vi "Write VariableGroupRingRef.vi"(8 "error in (no error)":errorcluster, 10 "VariableGroupRingRef":refnum<vi>, 11 "VMUI in":refnum<class "VMUI.lvclass">) -> (0 "error out":errorcluster, 3 "VMUI out":refnum<class "VMUI.lvclass">)   [LabVIEW 2013, in "VMUI.lvclass"]
uses:
  VMUI.lvclass
  VMUI.lvclass/VMUI.ctl
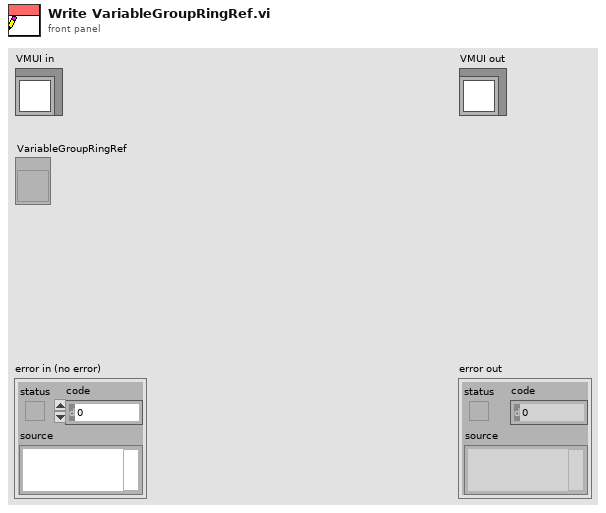
[diagram p1: front panel]
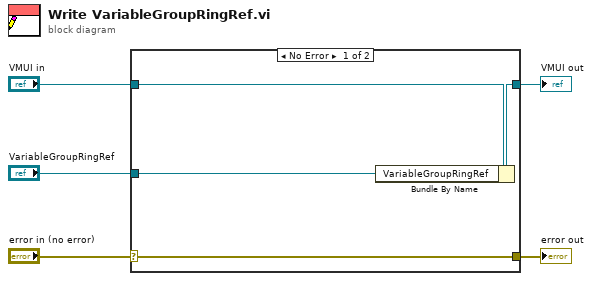
[diagram p0: block diagram]
diagram:
  n1 = case shown="No Error" "error in (no error)" {
    selector: "error in (no error)" -> [w9 w10]
    tunnel: [w9 w10] -> w4
    tunnel: [w7 w11] -> w2
    tunnel: "VMUI in" -> [w8 w11]
    tunnel: "VariableGroupRingRef" -> [w6 _]
    frame No Error {
      n2 = Bundle By Name(cluster=w8, "VariableGroupRingRef"=w6) -> (w7:refnum<class "VMUI.lvclass">)
    }
    frame Error {
    }
  }
  "error out" <- w4
  "VMUI out" <- w2
